vi "Pivot Controller.vi"(8 "error in":errorcluster) -> ()   [LabVIEW 2025]
doc: "This VI executes continuously carrying out the current operation and responding to updates or new operations. It will often contain the timing or control code that is difficult to place directly in TeleOp. This VI generally opens all sensors and motors and isolates the rest of the robot code from knowing how the operations are carried out."
uses:
  <vilib>/Rock Robotics/WPI/Framework/Completion Status.ctl
  Pivot Setpoints.ctl
  Pivot Operations.ctl
  <vilib>/Rock Robotics/WPI/ThirdParty/REV Robotics/REVLib/Typedef/SPARK PID Gains.ctl
  <vilib>/Rock Robotics/WPI/ThirdParty/REV Robotics/REVLib/Typedef/SPARK Feed Forward Gains.ctl
  <vilib>/Rock Robotics/WPI/ThirdParty/REV Robotics/REVLib/Typedef/Spark MAX Idle Mode.ctl
  <vilib>/Rock Robotics/WPI/ThirdParty/REV Robotics/REVLib/Typedef/Spark MAX Control Type.ctl
  <vilib>/Rock Robotics/WPI/ThirdParty/REV Robotics/REVLib/SubVI/Public/SPARK Open Brushless.vi
  <vilib>/Rock Robotics/WPI/ThirdParty/REV Robotics/REVLib/SubVI/Public/SPARK Configure Basic Idle Mode.vi
  Support Code/Globals.vi
  <vilib>/Rock Robotics/WPI/ThirdParty/REV Robotics/REVLib/SubVI/Public/SPARK Get Encoder Status Position.vi
  <vilib>/Rock Robotics/WPI/ThirdParty/REV Robotics/REVLib/SubVI/Public/SPARK Configure Closed Loop Gains.vi
  <vilib>/Rock Robotics/WPI/ThirdParty/REV Robotics/REVLib/SubVI/Public/SPARK Configure Power Current Limit.vi
  <vilib>/Rock Robotics/WPI/ThirdParty/REV Robotics/REVLib/SubVI/Public/SPARK Configure Closed Loop Output Range.vi
  <vilib>/Rock Robotics/Network Tables/NT Write Boolean.vi
panel:
  in  "Tolerance Retract":dbl=0.05
  in  "Tolerance Extend":dbl=0.05
  in  "Maximum Output":dbl=0.23
  in  "Minimum Output":dbl=-0.75
  in  "Retracted Setpoint":dbl=1.0
  in  "Extended Setpoint":dbl=23.0
  in  "Pivot  FF":T1
  in  "Pivot PID":T2={"kP"=0.35, "kI"=0.0, "kD"=12.0}
  in  "Interactive Values":T3
  out "Current\nCmd":string
  in  "Buttons":cluster{"Execute Cmd":bool, "Abort Cmd":bool}
  out "Command Timing":cluster{"Start Time (ms)":u32, "Iterations":i32}
  out "Status":T5
  # "Interactive Command: You may fill in the settings for a command\nand schedule it with the Execute button. You can observe and abort\nany command while fine tuning the code for the controller."
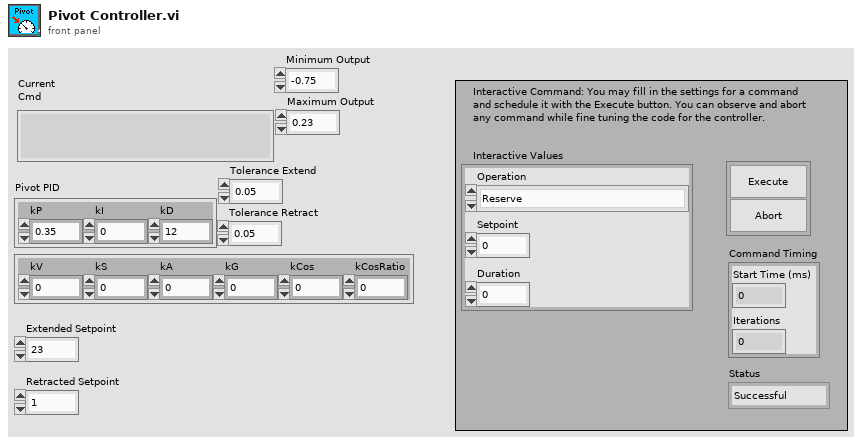
[diagram p1: front panel]
types:
  T1 = typedef "SPARK Feed Forward Gains.ctl" = cluster{"kV":dbl, "kS":dbl, "kA":dbl, "kG":dbl, "kCos":dbl, "kCosRatio":dbl}
  T2 = typedef "SPARK PID Gains.ctl" = cluster{"kP":dbl, "kI":dbl, "kD":dbl}
  T3 = typedef "Pivot Setpoints.ctl" = cluster{"Operation":T4, "Setpoint":dbl, "Duration":dbl}
  T4 = typedef "Pivot Operations.ctl" = enum16{"Reserve", "Read Current", "Retract Pivot", "Extend Pivot", "Reset Pivot", "Immediate", "Extend Pivot Auto", "Retract Pivot Auto"}
  T5 = typedef "Completion Status.ctl" = enum16{"Successful", "Aborted", "Incomplete"}
  T6 = typedef "Spark MAX Idle Mode.ctl" = enum16{"Coast", "Brake"}
  T7 = typedef "WPI_MotorControlDeviceRef.ctl" = cluster{"DeviceStatus":errorcluster, "Type":T8, "PWM":cluster{"PWM Channel":T9, "DeadBand":T10}, "CAN":cluster{"Device Number":u8, "SetOutput VI Ref":variant, "GetOutput VI Ref":variant, "Enable VI Ref":variant, "Disable VI Ref":variant, "Data":variant}, "Invert":bool, "DIO PWM":cluster{"PWM \"Enable\" Channel":T9, "DIOChannel":T11, "PWM Rate":dbl}}
  T8 = typedef "WPI_MotorControlType.ctl" = enum16{"PWM", "CAN", "DIO PWM"}
  T9 = typedef "FPGA_DIOPWMChannel.ctl" = enum8{"PWM 0", "PWM 1", "PWM 2", "PWM 3", "PWM 4", "PWM 5", "PWM 6", "PWM 7", "PWM 8", "PWM 9", "PWM MXP 0", "PWM MXP 1", "PWM MXP 2", "PWM MXP 3", "PWM MXP 4", "PWM MXP 5", "PWM MXP 6", "PWM MXP 7", "PWM MXP 8", "PWM MXP 9", "Invalid"}
  T10 = typedef "WPI_PWMDeadband.ctl" = cluster{"Name":string, "maxPositivePwm":i32, "minPositivePwm":i32, "centerPwm":i32, "maxNegativePwm":i32, "minNegativePwm":i32, "angularRange":u16}
  T11 = typedef "FPGA_DIOChannel.ctl" = enum8{"DIO 0", "DIO 1", "DIO 2", "DIO 3", "DIO 4", "DIO 5", "DIO 6", "DIO 7", "DIO 8", "DIO 9", "DIO MXP 0", "DIO MXP 1", "DIO MXP 2", "DIO MXP 3", "DIO MXP 4", "DIO MXP 5", "DIO MXP 6", "DIO MXP 7", "DIO MXP 8", "DIO MXP 9", "DIO MXP 10", "DIO MXP 11", "DIO MXP 12", "DIO MXP 13", "DIO MXP 14", "DIO MXP 15", "SPI Port CS1", "SPI Port CS2", "SPI Port CS3", "SPI Port MISO", "SPI Port MOSI", "Invalid"}
  T12 = typedef "Command Status Info.ctl" = cluster{"Name":string, "Status":T5, "notifier out":T13}
  T13 = typedef "Completion Notifier.ctl" = refnum<notifier>
  T14 = cluster{"Current Command":T3, "Command Timing":cluster{"Start Time (ms)":u32, "Iterations":i32}, "Command Arguments":cluster{"Command Info":T12, "Description":string, "Default Command":T3, "queue out":refnum<queue>, "Subsystem Name":string}}
  T15 = typedef "Spark MAX Control Type.ctl" = enum16{"Percent VBus", "Voltage", "Velocity", "Position", "Smart Motion", "Current", "Smart Velocity", "MAXMotion Position", "MAXMotion Velocity"}
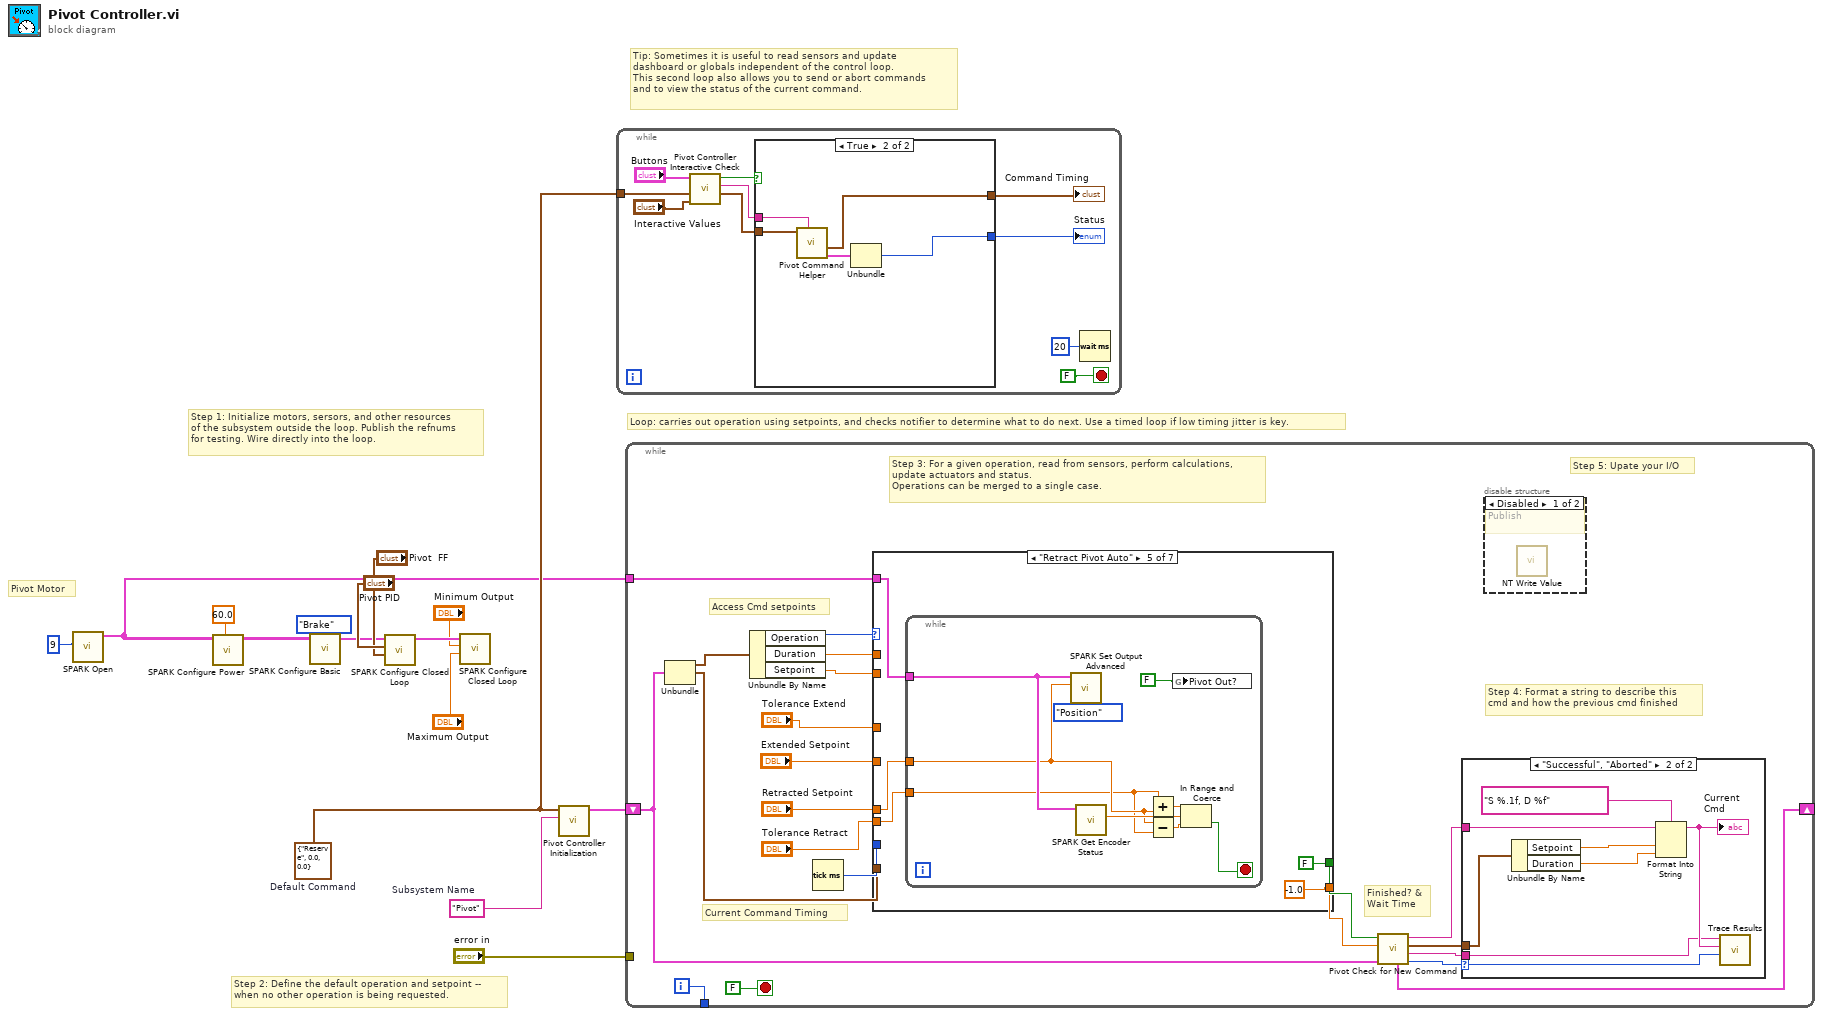
[diagram p0: block diagram]
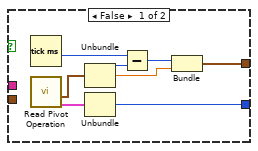
[diagram p2: hidden frame]
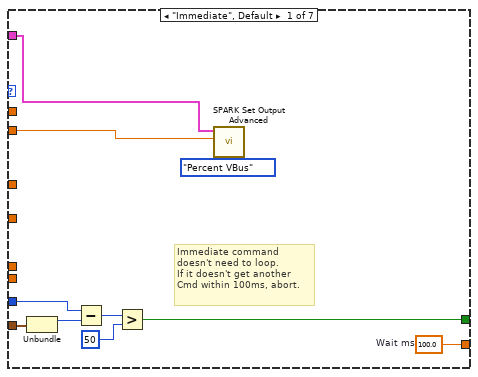
[diagram p5: hidden frame]
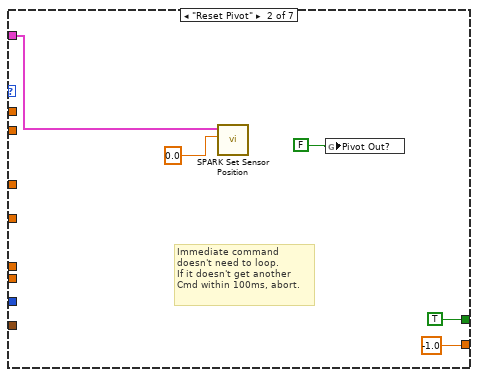
[diagram p6: hidden frame]
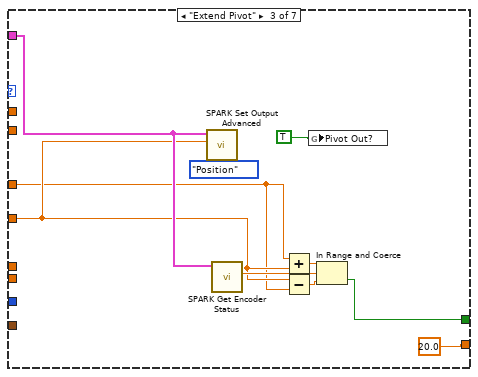
[diagram p7: hidden frame]
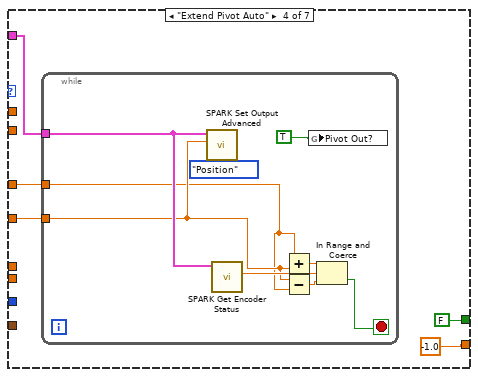
[diagram p8: hidden frame]
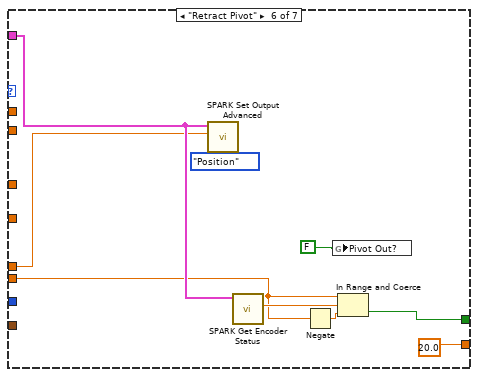
[diagram p9: hidden frame]
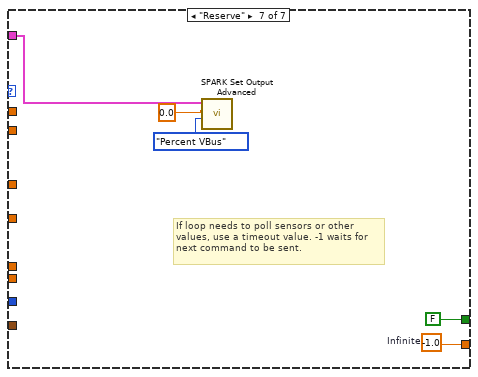
[diagram p10: hidden frame]
diagram:
  w10 = T3 {"Operation"=enum."Reserve", "Setpoint"=0.0, "Duration"=0.0}  # Default Command
  w11 = "Pivot"  # Subsystem Name
  # "Pivot Motor"
  # "Tip: Sometimes it is useful to read sensors and update\ndashboard or globals independent of the control loop.\nThis second loop also allows you to send or abort commands\nand to view the status of the current command."
  # "Step 2: Define the default operation and setpoint --\nwhen no other operation is being requested."
  # "Step 1: Initialize motors, sersors, and other resources\nof the subsystem outside the loop. Publish the refnums\nfor testing. Wire directly into the loop."
  # "Loop: carries out operation using setpoints, and checks notifier to determine what to do next. Use a timed loop if low timing jitter is key."
  n1 = call-poly <vilib>:"SPARK Open.vi"("Device Number"=u8 9) -> ("MotorControlDeviceRef"=w5:T7)  [unwired: 9 in, 1 out]
  n2 = call-poly <vilib>:"SPARK Configure Power.vi"("Current Limit A (100)"=sgl 60.0, "MotorControlDeviceRef in"=w5) -> ()  [unwired: 8 in, 2 out]
  n3 = call-poly <vilib>:"SPARK Configure Basic.vi"("Idle Mode"=Spark_MAX_Idle_Mode."Brake", "MotorControlDeviceRef in"=w5) -> ()  [unwired: 8 in, 2 out]
  n4 = call-poly <vilib>:"SPARK Configure Closed Loop.vi"("Feed Forward Gains"="Pivot  FF", "PID Gains"="Pivot PID", "MotorControlDeviceRef in"=w5) -> ("MotorControlDeviceRef out"=w3:T7)  [unwired: 7 in, 1 out]
  n5 = call-poly <vilib>:"SPARK Configure Closed Loop.vi"("Maximum Output"="Maximum Output", "Minimum Output"="Minimum Output", "MotorControlDeviceRef in"=w3) -> ()  [unwired: 7 in, 2 out]
  n6 = call "Pivot Controller Initialization.vi"("Subsystem Name"=w11, "Default Command"=w10) -> ("Current Command"=w12:T14)  [unwired: 9 in]
  n7 = while {
    tunnel: w10 -> [w20]
    stop <- FALSE stop-if-true
    n8 = call "Pivot Controller Interactive Check.vi"("Interactive Command in"="Interactive Values", "Default Command"=w20, "Buttons"="Buttons") -> ("Interactive Command out"=w17:T3, "Trace String"=w18:string, "Schedule"=w19:bool)  [unwired: 6 in]
    n9 = case shown="True" w19 {
      tunnel: [w31 w36] -> w16
      tunnel: w17 -> [_ w34]
      tunnel: [w27 w32] -> w15
      tunnel: w18 -> [_ w35]
      frame False {
        n10 = Tick Count (ms)() -> (millisecond timer value=w26:u32)
        n11 = call "Read Pivot Operation.vi"() -> ("Command Info"=w24:T12, "SubSystem Data"=w25:T3)  [unwired: 9 in, 1 out]
        n12 = Unbundle(w25) -> ("Operation"=w30:T4, "Setpoint"=w28:dbl)  [unwired: 1 out]
        n13 = Unbundle(w24) -> ("Status"=w31:T5)  [unwired: 2 out]
        n14 = Subtract(x=w26, y=w30) -> (x-y=w29:u32)
        n15 = Bundle(w29, "Setpoint"=w28) -> (w27:cluster{u32, "Setpoint":dbl})  [unwired: 1 in]
      }
      frame True {
        n16 = call "Pivot Command Helper.vi"("Description"=w35, "SubSystem Data"=w34) -> ("Command Info Out"=w33:T12, "Command Timing"=w32:cluster{"Start Time (ms)":u32, "Iterations":i32})  [unwired: 7 in, 1 out]
        n17 = Unbundle(w33) -> ("Status"=w36:T5)  [unwired: 2 out]
      }
    }
    "Status" <- w16
    "Command Timing" <- w15
    n18 = Wait (ms)(milliseconds to wait=u32 20) -> ()  [unwired: 1 out]
  }
  n19 = while {
    shift-right: [w49] -> _
    shift-left: w12 -> [w42]
    tunnel: [w56] -> _
    tunnel: "error in" -> [_]
    tunnel: w5 -> [w41]
    i -> [w56]
    stop <- FALSE stop-if-true
    # "Step 5: Upate your I/O"
    # "Step 4: Format a string to describe this\ncmd and how the previous cmd finished"
    # "Current Command Timing"
    # "Access Cmd setpoints"
    # "Finished? &\nWait Time"
    # "Step 3: For a given operation, read from sensors, perform calculations,\nupdate actuators and status.\nOperations can be merged to a single case."
    n20 = Unbundle(w42) -> ("Current Command"=w55:T3, "Command Timing"=w51:cluster{"Start Time (ms)":u32, "Iterations":i32})  [unwired: 1 out]
    n21 = Unbundle By Name(w55) -> ("Operation"=w54:T4, "Duration"=w53:dbl, "Setpoint"=w50:dbl)
    n22 = Tick Count (ms)() -> (millisecond timer value=w52:u32)
    n23 = case shown="\"Retract Pivot Auto\"" w54 {
      tunnel: [w75 -1.0 ("Infinite") 20.0 ("Infinite") -1.0 ("Infinite") -1.0 ("Infinite") 20.0 ("Infinite") w132] -> w47
      tunnel: [w69 TRUE ("ignore previous (F)") w85 FALSE ("ignore previous (F)") FALSE ("ignore previous (F)") w121 FALSE ("ignore previous (F)")] -> w48
      tunnel: w51 -> [w71 _ _ _ _ _ _]
      tunnel: w53 -> [_ _ _ _ _ _ _]
      tunnel: w52 -> [w70 _ _ _ _ _ _]
      tunnel: w50 -> [w67 _ _ _ _ _ _]
      tunnel: w41 -> [w68 w80 w87 w94 w108 w122 w130]
      tunnel: "Extended Setpoint" -> [_ _ w82 w92 _ _ _]
      tunnel: "Retracted Setpoint" -> [_ _ _ _ w106 w120 _]
      tunnel: "Tolerance Extend" -> [_ _ w81 w91 _ _ _]
      tunnel: "Tolerance Retract" -> [_ _ _ _ w105 w119 _]
      frame "Immediate", Default {
        w75 = 100.0  # Wait ms
        # "Immediate command\ndoesn't need to loop.\nIf it doesn't get another\nCmd within 100ms, abort."
        n24 = Unbundle(w71) -> ("Start Time (ms)"=w74:u32)  [unwired: 1 out]
        n25 = Subtract(x=w70, y=w74) -> (x-y=w73:u32)
        n26 = Greater?(x=w73, y=u8 50 ("Left Motor")) -> (0:w69:bool)
        n27 = call <vilib>:"SPARK Set Output Advanced.vi"("Control Mode"=Spark_MAX_Control_Type."Percent VBus", "Setpoint"=w67, "MotorControlDevRef"=w68) -> ()  [unwired: 7 in, 2 out]
      }
      frame "Reset Pivot" {
        # "Immediate command\ndoesn't need to loop.\nIf it doesn't get another\nCmd within 100ms, abort."
        n28 = call <vilib>:"SPARK Set Sensor Position.vi"("Position"=0.0, "MotorControlDeviceRef"=w80) -> ()  [unwired: 8 in, 2 out]
        n29 = global write "Globals.vi" "Pivot Out?"(FALSE ("Pivot Out?")) -> ()
      }
      frame "Extend Pivot" {
        n30 = call <vilib>:"SPARK Set Output Advanced.vi"("Control Mode"=Spark_MAX_Control_Type."Position", "Setpoint"=w82, "MotorControlDevRef"=w87) -> ()  [unwired: 7 in, 2 out]
        n31 = call-poly <vilib>:"SPARK Get Encoder Status.vi"("MotorControlDevRef in"=w87) -> ("Sensor Position"=w86:dbl)  [unwired: 7 in, 3 out]
        n32 = Add(x=w81, y=w82) -> (x+y=w84:dbl)
        n33 = Subtract(x=w82, y=w81) -> (x-y=w83:dbl)
        n34 = global write "Globals.vi" "Pivot Out?"(TRUE ("Pivot Out?")) -> ()
        n35 = In Range and Coerce(upper limit=w84, x=w86, lower limit=w83) -> (In Range?=w85:bool)  [unwired: 1 out]
      }
      frame "Extend Pivot Auto" {
        n36 = while {
          tunnel: w94 -> [w102]
          tunnel: w92 -> [w97]
          tunnel: w91 -> [w96]
          stop <- w98 stop-if-true
          n37 = call <vilib>:"SPARK Set Output Advanced.vi"("Control Mode"=Spark_MAX_Control_Type."Position", "Setpoint"=w97, "MotorControlDevRef"=w102) -> ()  [unwired: 7 in, 2 out]
          n38 = call-poly <vilib>:"SPARK Get Encoder Status.vi"("MotorControlDevRef in"=w102) -> ("Sensor Position"=w101:dbl)  [unwired: 7 in, 3 out]
          n39 = Add(x=w96, y=w97) -> (x+y=w100:dbl)
          n40 = Subtract(x=w97, y=w96) -> (x-y=w99:dbl)
          n41 = global write "Globals.vi" "Pivot Out?"(TRUE ("Pivot Out?")) -> ()
          n42 = In Range and Coerce(upper limit=w100, x=w101, lower limit=w99) -> (In Range?=w98:bool)  [unwired: 1 out]
        }
      }
      frame "Retract Pivot Auto" {
        n43 = while {
          tunnel: w108 -> [w116]
          tunnel: w106 -> [w111]
          tunnel: w105 -> [w110]
          stop <- w112 stop-if-true
          n44 = call <vilib>:"SPARK Set Output Advanced.vi"("Control Mode"=Spark_MAX_Control_Type."Position", "Setpoint"=w111, "MotorControlDevRef"=w116) -> ()  [unwired: 7 in, 2 out]
          n45 = call-poly <vilib>:"SPARK Get Encoder Status.vi"("MotorControlDevRef in"=w116) -> ("Sensor Position"=w115:dbl)  [unwired: 7 in, 3 out]
          n46 = Add(x=w110, y=w111) -> (x+y=w114:dbl)
          n47 = Subtract(x=w111, y=w110) -> (x-y=w113:dbl)
          n48 = global write "Globals.vi" "Pivot Out?"(FALSE ("Pivot Out?")) -> ()
          n49 = In Range and Coerce(upper limit=w114, x=w115, lower limit=w113) -> (In Range?=w112:bool)  [unwired: 1 out]
        }
      }
      frame "Retract Pivot" {
        n50 = call <vilib>:"SPARK Set Output Advanced.vi"("Control Mode"=Spark_MAX_Control_Type."Position", "Setpoint"=w120, "MotorControlDevRef"=w122) -> ()  [unwired: 7 in, 2 out]
        n51 = call-poly <vilib>:"SPARK Get Encoder Status.vi"("MotorControlDevRef in"=w122) -> ("Sensor Position"=w124:dbl)  [unwired: 7 in, 3 out]
        n52 = Negate(x=w119) -> (-x=w123:dbl)
        n53 = global write "Globals.vi" "Pivot Out?"(FALSE ("Pivot Out?")) -> ()
        n54 = In Range and Coerce(upper limit=w119, x=w124, lower limit=w123) -> (In Range?=w121:bool)  [unwired: 1 out]
      }
      frame "Reserve" {
        w132 = -1.0  # Infinite
        # "If loop needs to poll sensors or other\nvalues, use a timeout value. -1 waits for\nnext command to be sent."
        n55 = call <vilib>:"SPARK Set Output Advanced.vi"("Control Mode"=Spark_MAX_Control_Type."Percent VBus", "Setpoint"=0.0, "MotorControlDevRef"=w130) -> ()  [unwired: 7 in, 2 out]
      }
    }
    n56 = call "Pivot Check for New Command.vi"("Current Command"=w42, "Wait time (ms)"=w47, "Finished?"=w48) -> ("Completion"=w43:T5, "Subsystem Name"=w44:string, "Current Command"=w45:T3, "Initial Trace String"=w46:string, "NextCommand"=w49:T14)  [unwired: 4 in]
    n57 = case shown="\"Successful\", \"Aborted\"" w43 {
      selector: w43 -> [_ w65]
      tunnel: w46 -> [_ w61]
      tunnel: w45 -> [_ w62]
      tunnel: w44 -> [_ w58]
      frame "Incomplete", Default {
        # "Continuing current command"
      }
      frame "Successful", "Aborted" {
        # "Report and setup for next command"
        n58 = Unbundle By Name(w62) -> ("Setpoint"=w64:dbl, "Duration"=w59:dbl)
        n59 = Format Into String(format string="S %.1f, D %f", initial string=w61, w64, w59) -> (resulting string=w60:string)  [unwired: 1 in, 1 out]
        "Current\nCmd" <- w60
        n60 = call <vilib>:"Trace Results.vi"("Status of previous command"=w65, "Description"=w60, "Subsystem"=w58) -> ()  [unwired: 9 in]
      }
    }
    n61 = disable-structure shown="Disabled" {
      frame Disabled {
        # "Publish"
        n62 = call-poly <vilib>:"NT Write Value.vi"() -> ()  [unwired: 11 in, 1 out]
      }
      frame Enabled {
      }
    }
  }
